vi "SetValue.vi"(8 "error in":errorcluster, 10 "Value":string, 11 "NonEmptyString in":refnum<class "NonEmptyString.lvclass">) -> (0 "error out":errorcluster, 3 "NonEmptyString out":refnum<class "NonEmptyString.lvclass">)   [LabVIEW 2021, in "ProligentXMLGenerator.lvlib" / "NonEmptyString.lvclass"]
uses:
  NonEmptyString.lvclass
  NonEmptyString.lvclass/NonEmptyString.ctl
  String/String.lvclass
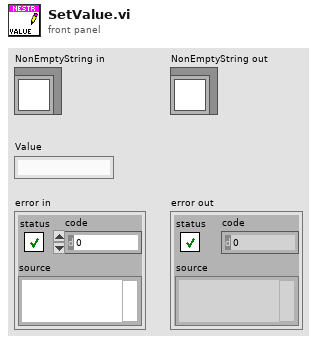
[diagram p1: front panel]
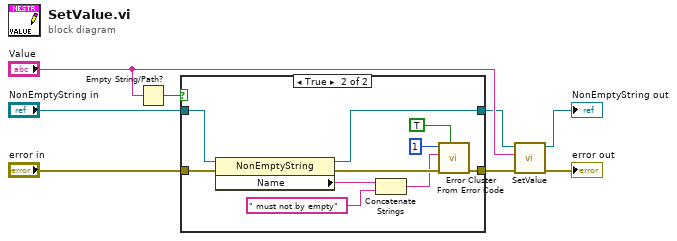
[diagram p0: block diagram]
diagram:
  n1 = Empty String/Path?(string/path="Value") -> (empty?=w6:bool)
  n2 = case shown="True" w6 {
    tunnel: "NonEmptyString in" -> [w10 w16]
    tunnel: [w10 w12] -> w2
    tunnel: "error in" -> [w9 w19]
    tunnel: [w9 w18] -> w5
    frame False {
    }
    frame True {
      n3 = property on="Property Node" class="NonEmptyString"(reference=w16, error in=w19) -> (reference out=w12:refnum<class "NonEmptyString.lvclass">, error out=w17:errorcluster, "Name"=w15:string)
      n4 = Concatenate Strings(w15, " must not by empty" ("string")) -> (w14:string)
      n5 = call <vilib>:"Error Cluster From Error Code.vi"("show call chain? (False)"=TRUE, "error in (no error)"=w17, "error message (\"\")"=w14, "error code (0)"=1) -> ("error out"=w18:errorcluster)  [unwired: 5 in]
    }
  }
  n6 = call-parent "SetValue.vi"("error in"=w5, "Value"="Value", "String in"=w2) -> ("error out"=→"error out":errorcluster, "String out"=→"NonEmptyString out":refnum<class "NonEmptyString.lvclass">)  [unwired: 7 in]
